vi "ToStrings.vi"(1 "Things":refnum<class "WebSocket.lvclass">[](array[class])) -> (0 "String":string)   [LabVIEW 2017, in "WebSocket.lvclass"]
uses:
  WebSocket.lvclass
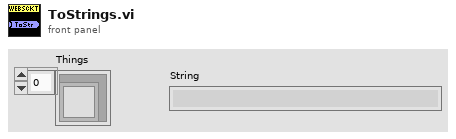
[diagram p1: front panel]
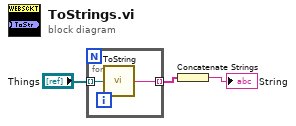
[diagram p0: block diagram]
diagram:
  n1 = for {
    tunnel: "Things" -> [w5] mode=indexing
    tunnel: [w4] -> w2 mode=indexing
    n2 = call "ToString.vi"("WebSocket"=w5) -> ("String"=w4:string)
  }
  n3 = Concatenate Strings(w2) -> (→"String":string)
